vi "Status Update.vi"(8 "error in (no error)":errorcluster, 11 "Autosampler in":refnum<class "Autosampler.lvclass">) -> (0 "error out":errorcluster, 2 "Autosampler Status":T1, 3 "Autosampler out":refnum<class "Autosampler.lvclass">)   [LabVIEW 2023, in "Autosampler.lvlib" / "Autosampler.lvclass"]
uses:
  Autosampler.lvclass
  Autosampler.lvclass/Autosampler.ctl
  Application Messages/Autosampler Status Update Msg/Autosampler Status Update Msg.lvclass
  <vilib>/ActorFramework/Message Enqueuer/Message Enqueuer.lvclass
  <vilib>/ActorFramework/Actor/Actor.lvclass
  Autosampler Status.ctl
  Autosampler.lvlib
  Autosampler State.ctl
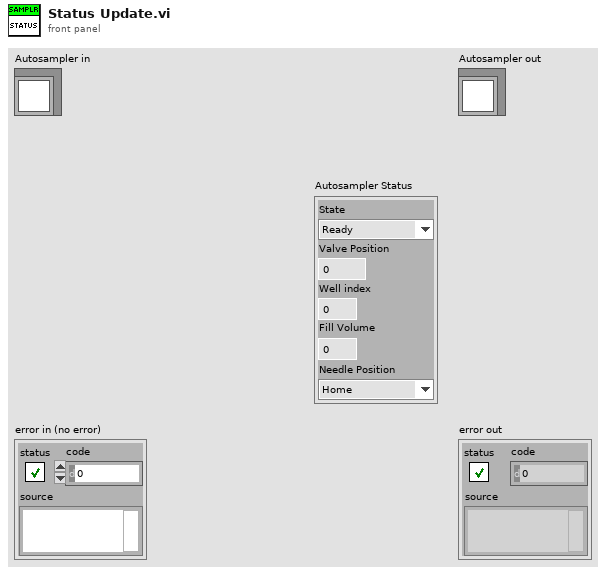
[diagram p1: front panel]
types:
  T1 = typedef "Autosampler.lvlib/Autosampler Status.ctl" = cluster{"State":T2, "Valve Position":u16, "Well index":u16, "Fill Volume":u16, "Needle Position":enum16{"Home", "Well", "Wash Port"}}
  T2 = typedef "Autosampler.lvlib/Autosampler State.ctl" = enum16{"Ready", "Injection", "Washing", "Shaking", "Getting Ready", "Error"}
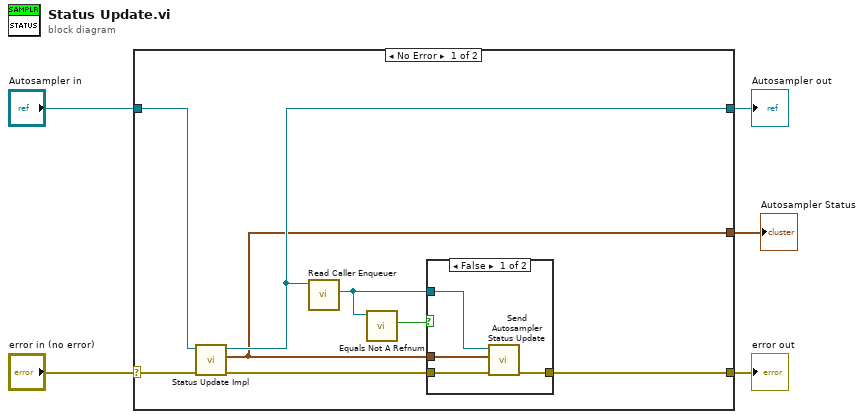
[diagram p0: block diagram]
diagram:
  n1 = case shown="No Error" "error in (no error)" {
    selector: "error in (no error)" -> [w12 w20]
    tunnel: [w13 w20] -> w4
    tunnel: [w10 w19] -> w2
    tunnel: "Autosampler in" -> [w11 w19]
    tunnel: [w9 _] -> w1
    frame No Error {
      n2 = call-dynamic "Status Update Impl.vi"("error in (no error)"=w12, "Autosampler in"=w11) -> ("error out"=w8:errorcluster, "Autosampler Status"=w9:T1, "Autosampler out"=w10:refnum<class "Autosampler.lvclass">)  [unwired: 7 in]
      n3 = call <vilib>:"Read Caller Enqueuer.vi"("Actor"=w10) -> ("Caller Enqueuer"=w7:refnum<class "Message Enqueuer.lvclass">)  [unwired: 10 in]
      n4 = call <vilib>:"Equals Not A Refnum.vi"("Message Enqueuer"=w7) -> ("Not a refnum?"=w6:bool)  [unwired: 10 in]
      n5 = case shown="False" w6 {
        tunnel: [w17 w18] -> w13
        tunnel: w9 -> [w16 _]
        tunnel: w8 -> [w15 w18]
        tunnel: w7 -> [w14 _]
        frame False {
          n6 = call "Send Autosampler Status Update.vi"("error in (no error)"=w15, "Autosampler Status"=w16, "Message Enqueuer"=w14) -> ("error out"=w17:errorcluster)  [unwired: 7 in, 1 out]
        }
        frame True {
          # "root actor.\nno parent."
        }
      }
    }
    frame Error {
    }
  }
  "error out" <- w4
  "Autosampler out" <- w2
  "Autosampler Status" <- w1
